vi "LLB - Controls.vi"(7 "Msg Chain":string, 8 "error in (no error)":errorcluster {"code" format="Error %.0f"}, 10 "LLBs":refnum<class "LLB Documentation.lvclass">[](array[class]), 11 "VIDoc Printer - Confluence In":refnum<class "VIDoc Printer - Confluence.lvclass">) -> (0 "error out":errorcluster {"code" format="Error %.0f"}, 3 "VIDoc Printer - Confluence Out":refnum<class "VIDoc Printer - Confluence.lvclass">)   [LabVIEW 2023, in "VIDoc Printer - Confluence.lvlib" / "VIDoc Printer - Confluence.lvclass"]
uses:
  VIDoc Printer - Confluence.lvclass
  C:/projects/DMC/Tooling/Git-Action-Service/Source/Documentation Generation/Printers/Printer/VIDoc Printer.lvclass
  Parsing/LLB Documentation/LLB Documentation.lvclass
  Parsing/LLB Documentation/LLB Documentation.lvclass/LLB Documentation.ctl
  Printer/VIDoc Printer.lvclass/VIDoc Printer.ctl
  Parsing/TypeDefs/VI Type Extended Enum.ctl
  Settings/Printer Settings/Scope Settings.ctl
  Confluence Formatting/Types/Format Combo Box.ctl
  VIDoc Printer - Confluence.lvclass/VIDoc Printer - Confluence.ctl
  Accessors/Get VI Controls Expand.vi
  Printer/Accessors/Get LLB Settings - Controls Detail Level.vi
  Parsing/LLB Documentation/Get LLB Methods.vi
  Parsing/LLB Documentation/Get Name.vi
  Printer/VIDoc Printer.lvclass
  UI Interaction/UI Interaction.lvclass
  Parsing/VIDoc Parsing.lvlib
  Settings/Printer Settings/Printer Settings.lvclass
  Confluence Formatting/Confluence Formatting.lvlib
  C:/projects/DMC/Tooling/Git-Action-Service/Source/Documentation Generation/Printers/Confluence Printer/VIDoc Printer - Confluence.lvclass
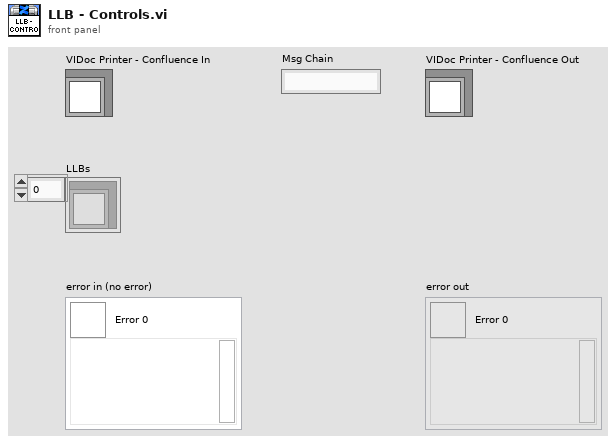
[diagram p1: front panel]
types:
  T1 = typedef "VIDoc Printer.lvlib/Printer Settings.lvclass/Scope Settings.ctl" = cluster{"Public":bool, "Protected":bool, "Community":bool, "Private":bool, "Unknown":bool}
  T2 = typedef "VIDoc Parsing.lvlib/VI Type Extended Enum.ctl" = enum16{"Unknown", "Class Method", "Class Accessor Get", "Class Accessor Set", "Class Control", "Library Method", "Library Control", "VI", "Control"}
  T3 = typedef "Confluence Formatting.lvlib/Format Combo Box.ctl" = string
  T4 = typedef "VIDoc Parsing.lvlib/Method Spec Cluster.ctl" = cluster{"VI Type Ext":T2, "Name":string, "Path":path, "Get Conpane Image":T5, "Description":string, "Get Library Access Scope":enum32{"invalid scope", "public", "private", "protected", "community"}, "Dispatch":T6, "ContainsCompiledCode":bool, "Exec.IsReentrant":bool, "Exec.ReentrancyType":enum16{"Share clones between instances", "Preallocate clone for each instance"}, "ExecInlining":bool, "ExecInlineIfPossible":bool, "Auto Err Handling":bool, "CodeComplexity":sgl, "Bookmark Tags":string[], "Control VI Type":enum32{"not a control VI", "control", "typedef", "strict typedef"}, "Controls":T7[], "VI Type":enum32{"invalid VI type", "Standard VI", "Control VI", "Global VI", "Polymorphic VI", "Configuration VI", "SubSystem", "Facade VI", "Method VI", "Statechart Diagram VI"}, "Minimum Size":T9, "Front Panel Window:Title":string, "Front Panel Window:Behavior":enum32{"Invalid", "Default", "Floating", "Floating/Auto-Hide", "Modal"}, "Front Panel Window:Closeable":bool, "Must Override":bool, "Must Use Parent Implementation":bool, "VI Icon":T5, "Front Panel":T5, "History:Revision Number":u32, "Metrics:Total Data Size":u32, "Execution:Allow Debugging":bool, "Execution:Preferred Exec System":enum32{"invalid execution system", "user interface", "standard", "instrument i/o", "data acquisition", "other 1", "other 2", "same as caller"}, "Execution:Priority":enum32{"invalid priority", "background priority", "normal priority", "above normal priority", "high priority", "time critical priority", "subroutine"}, "BM Tag Text":string[], "Block Diagram":T5, "Structure Tree":T10[]}
  T5 = typedef "imagedata.ctl" = cluster{"image type":i32, "image depth":i32, "image":u8[], "mask":u8[], "colors":u32[], "Rectangle":cluster{"left":i16, "top":i16, "right":i16, "bottom":i16}}
  T6 = typedef "VIDoc Parsing.lvlib/Class Dispatch Type Enum.ctl" = enum16{"None", "Static", "Dynamic"}
  T7 = typedef "VIDoc Parsing.lvlib/Controls Info Cluster.ctl" = cluster{"Name":string, "Description":string, "Data Type":string, "Tip Strip":string, "UID":i32, "Image Data":T5, "ToggleKeyBind":T8, "Raw Label":string, "Raw Caption":string}
  T8 = typedef "LVKeyTypeDef.ctl" = cluster{"Focus":bool, "Control":bool, "Shift":bool, "Key":string}
  T9 = typedef "LVPointTypeDef.ctl" = cluster{"Horizontal":i16, "Vertical":i16}
  T10 = typedef "VIDoc Parsing.lvlib/Structure Reporter.lvlib/Tree Cluster.ctl" = cluster{"Object Class Name":string, "Labels":string[], "Child Tag":string, "Item Indent":i32, "Child Only?":bool, "Glyph Index":i32}
  T11 = typedef "VIDoc Printer.lvlib/Printer Settings.lvclass/Detail Level Enum.ctl" = enum16{"None", "Minimal", "Standard", "Full"}
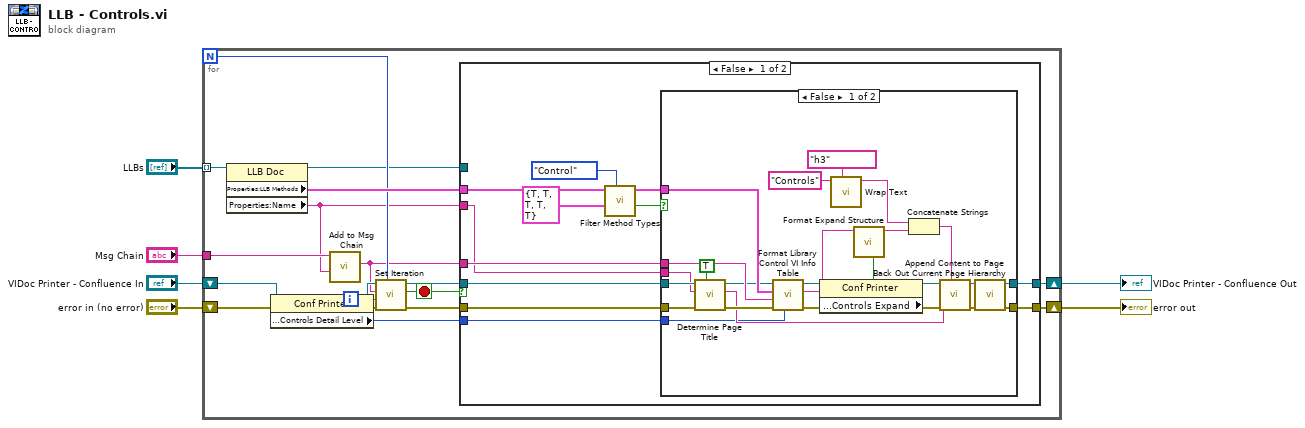
[diagram p0: block diagram]
diagram:
  n1 = for {
    N -> [w17]
    shift-right: [w22] -> w2
    shift-left: "error in (no error)" -> [w20]
    shift-right: [w23] -> w1
    shift-left: "VIDoc Printer - Confluence In" -> [w10]
    tunnel: "LLBs" -> [w24] mode=indexing
    tunnel: "Msg Chain" -> [w15]
    i -> [w16]
    stop <- w13 stop-if-true
    n2 = property class="LLB Doc"(reference=w24) -> (reference out=w12:refnum<class "LLB Documentation.lvclass">, "Properties:LLB Methods"=w21:T4[], "Properties:Name"=w14:string)  [unwired: 1 in, 1 out]
    n3 = property class="Conf Printer"(reference=w10, error in=w20) -> (reference out=w9:refnum<class "VIDoc Printer - Confluence.lvclass">, error out=w11:errorcluster, "Properties:Settings:LLBs:Controls Detail Level"=w7:T11)
    n4 = call "Add to Msg Chain.vi"("New"=w14, "Msg Chain in"=w15) -> ("Msg Chain out"=w8:string)  [unwired: 9 in]
    n5 = call "Set Iteration.vi"("Progress Max"=w17, "error in (no error)"=w11, "Progress Value"=w16, "Message (No Message Update)"=w8, "VIDoc Printer In"=w9) -> ("error out"=w18:errorcluster, "Abort?"=w13:bool, "VIDoc Printer Out"=w19:refnum<class "VIDoc Printer - Confluence.lvclass">)  [unwired: 4 in]
    n6 = case shown="False" w13 {
      tunnel: [w36 w63] -> w23
      tunnel: [w35 w64] -> w22
      tunnel: w21 -> [w30 _]
      tunnel: w19 -> [w33 w63]
      tunnel: w18 -> [w34 w64]
      tunnel: w14 -> [w31 _]
      tunnel: w12 -> [_ _]
      tunnel: w8 -> [w32 _]
      tunnel: w7 -> [w26 _]
      frame False {
        n7 = call "Filter Method Types.vi"("VI Type to filter for"=VI_Type_Extended_Enum."Control" ("y"), "Scope"=T1 {"Public"=TRUE, "Protected"=TRUE, "Community"=TRUE, "Private"=TRUE, "Unknown"=TRUE}, "Methods"=w30) -> ("All Filtered?"=w28:bool, "Filtered Methods"=w29:T4[])  [unwired: 6 in, 1 out]
        n8 = case shown="False" w28 {
          tunnel: [w43 w62] -> w36
          tunnel: [w45 w61] -> w35
          tunnel: w34 -> [w48 w61]
          tunnel: w33 -> [w50 w62]
          tunnel: w32 -> [w53 _]
          tunnel: w29 -> [w51 _]
          tunnel: w31 -> [w41 _]
          tunnel: w26 -> [w40 _]
          frame False {
            n9 = call "Determine Page Title.vi"("Update Current Page (F)"=TRUE, "error in (no error)"=w48, "Name"=w41, "VIDoc Printer - Confluence In"=w50) -> ("error out"=w47:errorcluster, "Page Title"=w42:string, "VIDoc Printer - Confluence Out"=w49:refnum<class "VIDoc Printer - Confluence.lvclass">)  [unwired: 4 in, 1 out]
            n10 = call "Format Library Control VI Info Table.vi"("Methods"=w40, "Error in"=w47, "Msg Chain"=w53, "VI Info Array"=w51, "VIDoc Printer - Confluence In"=w49) -> ("Error out"=w55:errorcluster, "Table String"=w52:string, "VIDoc Printer - Confluence Out"=w54:refnum<class "VIDoc Printer - Confluence.lvclass">)  [unwired: 4 in]
            n11 = property class="Conf Printer"(reference=w54) -> (reference out=w38:refnum<class "VIDoc Printer - Confluence.lvclass">, "Properties:Expand?:VI:Controls Expand"=w37:bool)  [unwired: 1 in, 1 out]
            n12 = call "Wrap Text.vi"("Formatting"=T3 "h3", "String"="Controls") -> ("Wrapped String"=w57:string)  [unwired: 8 in, 1 out]
            n13 = call "Format Expand Structure.vi"("Enable? (T)"=w37, "Content"=w52) -> ("Expand String"=w39:string)  [unwired: 8 in, 1 out]
            n14 = Concatenate Strings(w57, w39) -> (w56:string)
            n15 = call "Append Content to Page.vi"("Page Content"=w56, "error in (no error)"=w55, "Page Title"=w42, "VIDoc Printer - Confluence In"=w38) -> ("error out"=w60:errorcluster, "VIDoc Printer - Confluence Out"=w44:refnum<class "VIDoc Printer - Confluence.lvclass">)  [unwired: 6 in]
            n16 = call "Back Out Current Page Hierarchy.vi"("error in (no error)"=w60, "VIDoc Printer - Confluence In"=w44) -> ("error out"=w45:errorcluster, "VIDoc Printer - Confluence Out"=w43:refnum<class "VIDoc Printer - Confluence.lvclass">)  [unwired: 8 in]
          }
          frame True {
          }
        }
      }
      frame True {
      }
    }
  }
  "error out" <- w2
  "VIDoc Printer - Confluence Out" <- w1
